vi "Write TDMS Ref.vi"(8 "error in (no error)":errorcluster, 10 "TDMS Ref":refnum<k34>, 11 "TDMS in":refnum<class "TDMS.lvclass">) -> (0 "error out":errorcluster, 3 "TDMS out":refnum<class "TDMS.lvclass">)   [LabVIEW 2019, in "TDMS.lvlib" / "TDMS.lvclass"]
uses:
  TDMS.lvclass
  TDMS.lvclass/TDMS.ctl
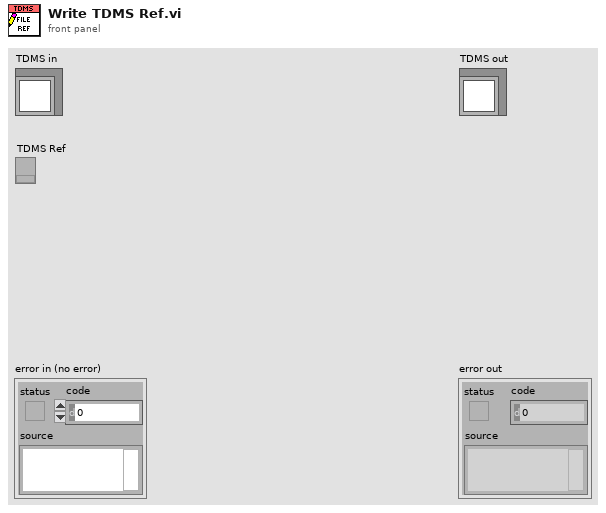
[diagram p1: front panel]
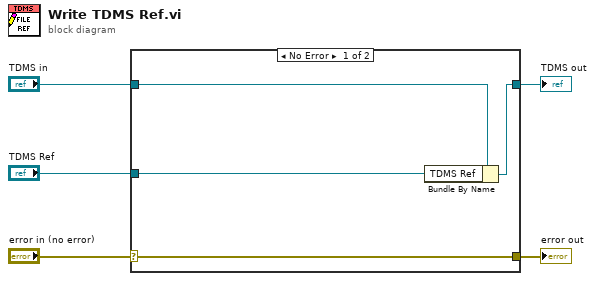
[diagram p0: block diagram]
diagram:
  n1 = case shown="No Error" "error in (no error)" {
    selector: "error in (no error)" -> [w9 w10]
    tunnel: [w9 w10] -> w4
    tunnel: [w7 w11] -> w2
    tunnel: "TDMS in" -> [w8 w11]
    tunnel: "TDMS Ref" -> [w6 _]
    frame No Error {
      n2 = Bundle By Name(cluster=w8, "TDMS Ref"=w6) -> (w7:refnum<class "TDMS.lvclass">)
    }
    frame Error {
    }
  }
  "error out" <- w4
  "TDMS out" <- w2
